vi "Open SequenceFile.vi"(7 "File Load Options":T1={"Use Search Dirs? (T)"=TRUE, "Conflict as Error? (T)"=TRUE, "Check Station Model? (F)"=FALSE, "Preload Modules? (T)"=TRUE, "Skip Load Callback? (F)"=FALSE, "Reload if Loaded? (F)"=FALSE}, 8 "error in (no error)":errorcluster, 9 "Current Seq File (None)":refnum<class "SequenceFile.lvclass">, 10 "File Path":path, 11 "Engine in":refnum<class "Engine.lvclass">) -> (0 "error out":errorcluster, 2 "SequenceFile":refnum<class "SequenceFile.lvclass">, 3 "Engine out":refnum<class "Engine.lvclass">)   [LabVIEW 2020, in "TSnax.lvlib" / "Engine.lvclass"]
uses:
  Engine.lvclass
  Engine.lvclass/Engine.ctl
  SequenceFile/SequenceFile.lvclass
  Open SequenceFile Response.ctl
  File Load Options.ctl
  TSnax.lvlib
  Open SequenceFile Request.ctl
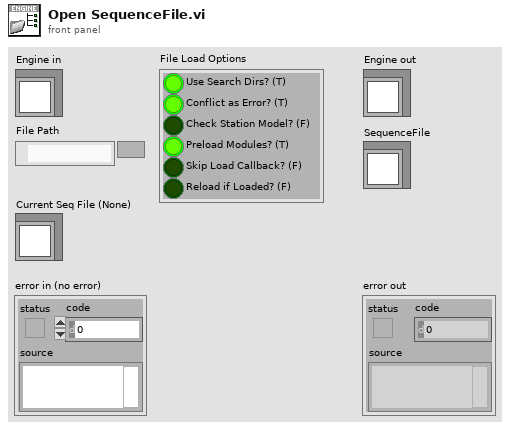
[diagram p1: front panel]
types:
  T1 = typedef "TSnax.lvlib/File Load Options.ctl" = cluster{"Use Search Dirs? (T)":bool, "Conflict as Error? (T)":bool, "Check Station Model? (F)":bool, "Preload Modules? (T)":bool, "Skip Load Callback? (F)":bool, "Reload if Loaded? (F)":bool}
  T2 = typedef "TSnax.lvlib/Engine.lvclass/Open SequenceFile Request.ctl" = cluster{"File Path":path, "File Load Options":T1, "Current SeqFile":refnum<class "SequenceFile.lvclass">, "Notifier":refnum<notifier>}
  T3 = typedef "TSnax.lvlib/Engine.lvclass/Open SequenceFile Response.ctl" = cluster{"SequenceFile":refnum<class "SequenceFile.lvclass">, "Error":errorcluster}
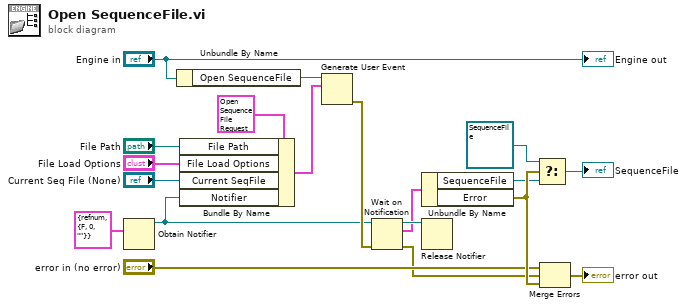
[diagram p0: block diagram]
diagram:
  n1 = Obtain Notifier(notification data type=T3 {"SequenceFile"=refnum, "Error"={"status"=FALSE, "code"=0, "source"=""}} ("Open SequenceFile Response")) -> (notifier out=w8:refnum<notifier>)  [unwired: 3 in, 2 out]
  n2 = Unbundle By Name("Engine in") -> ("Open SequenceFile"=w14:refnum<user-event>)
  n3 = Bundle By Name(cluster=T2 {"File Path"=path "", "File Load Options"={"Use Search Dirs? (T)"=TRUE, "Conflict as Error? (T)"=TRUE, "Check Station Model? (F)"=FALSE, "Preload Modules? (T)"=TRUE, "Skip Load Callback? (F)"=FALSE, "Reload if Loaded? (F)"=FALSE}, "Current SeqFile"=refnum, "Notifier"=refnum} ("event data"), "File Path"="File Path", "File Load Options"="File Load Options", "Current SeqFile"="Current Seq File (None)", "Notifier"=w8) -> (w9:T2)
  n4 = Generate User Event(user event=w14, event data cluster=w9) -> (error out=w18:errorcluster)  [unwired: 2 in, 1 out]
  n5 = Wait on Notification(notifier=w8, error in (no error)=w18) -> (notifier out=w7:refnum<notifier>, notification=w4:T3, error out=w5:errorcluster)  [unwired: 2 in, 1 out]
  n6 = Unbundle By Name(w4) -> ("SequenceFile"=w3:refnum<class "SequenceFile.lvclass">, "Error"=w19:errorcluster)
  n7 = Release Notifier(notifier=w7) -> ()  [unwired: 2 in, 3 out]
  n8 = Select(t=refnum<class "SequenceFile.lvclass"> refnum, s=w19, f=w3) -> (s? t:f=→"SequenceFile":refnum<class "SequenceFile.lvclass">)
  n9 = Merge Errors("error in (no error)", w5, w19) -> (→"error out":errorcluster)
  "Engine out" <- "Engine in"
